vi "WIFI_disconnectOne.vi"(8 "错误输入":errorcluster caption="错误输入（无错误）", 11 "WIFI_Name":string) -> (0 "error out":errorcluster caption="错误输出", 3 "standard output  2":string caption="标准输出")   [LabVIEW 2013]
uses:
  <vilib>/Utility/sysdir.llb/System Directory Type.ctl
panel:
  out "system directory":path caption="系统目录"
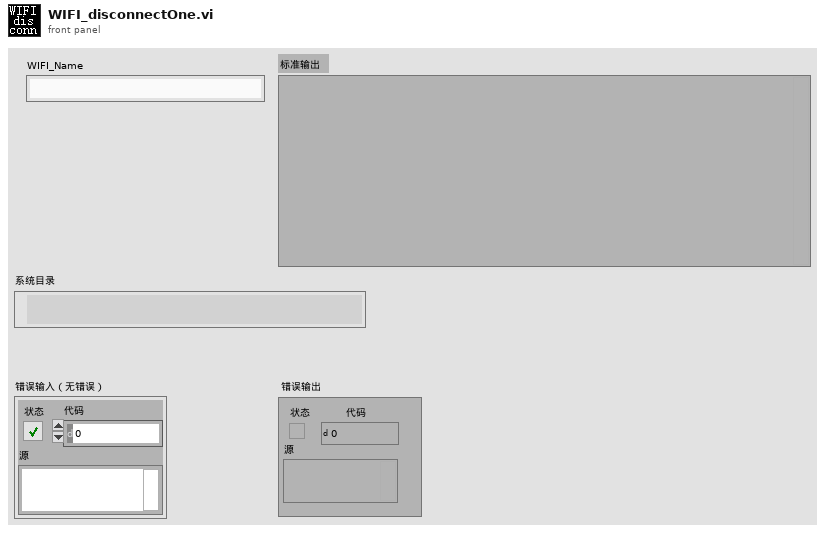
[diagram p1: front panel]
types:
  T1 = typedef "System Directory Type.ctl" = i32
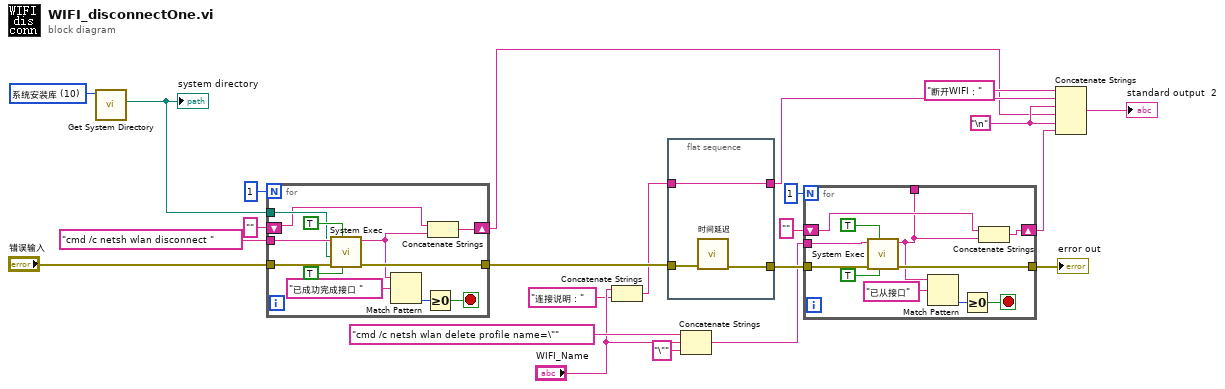
[diagram p0: block diagram]
diagram:
  w10 = "\n"
  w23 = T1 10 items=["用户目录"=0, "用户桌面"=1, "用户文档"=2, "用户应用程序数据"=3, "用户设置"=4, "用户临时目录"=5, "公共文档"=6, "公共应用程序数据"=7, "公共设置"=8, "公共缓存"=13, "系统核心库"=9, "系统安装库"=10, "应用程序文件"=11, "启动盘根目录"=12] ("system directory type")
  n1 = call <vilib>:"Get System Directory.vi"("system directory type"=w23) -> ("system directory"=w19:path)  [unwired: 10 in]
  "system directory" <- w19
  n2 = for {
    N: 1 -> [_]
    tunnel: "cmd /c netsh wlan disconnect " ("command line") -> [w33]
    tunnel: "错误输入" -> [w32]
    tunnel: [w31] -> w20
    tunnel: w19 -> [w30]
    shift-right: [w26] -> w2
    shift-left: "" -> [w25]
    stop <- w27 stop-if-true
    n3 = call <vilib>:"System Exec.vi"("run minimized? (F)"=TRUE, "wait until completion? (T)"=TRUE, "error in (no error)"=w32, "working directory"=w30, "command line"=w33) -> ("error out"=w31:errorcluster, "standard output"=w24:string)  [unwired: 3 in, 2 out]
    n4 = Match Pattern(string=w24, regular expression="已成功完成接口 " ("command line")) -> (offset past match=w28:i32)  [unwired: 1 in, 3 out]
    n5 = Greater Or Equal To 0?(x=w28) -> (x >= 0?=w27:bool)
    n6 = Concatenate Strings(w25, w24) -> (w26:string)
  }
  n7 = Concatenate Strings("WIFI_Name", "连接说明：" ("字符串")) -> (w13:string)
  n8 = flat-sequence {
    tunnel: w20 -> [w38]
    tunnel: [w37] -> w7
    tunnel: [w36] -> w11
    tunnel: w13 -> [w36]
    frame #0 {
      n9 = call "时间延迟"("error in (no error)"=w38) -> ("error out"=w37:errorcluster)  [unwired: 10 in]
    }
  }
  n10 = Concatenate Strings("cmd /c netsh wlan delete profile name=\"" ("command line"), "WIFI_Name", "\"" ("字符串")) -> (w1:string)
  n11 = for {
    N: 1 -> [_]
    tunnel: [w47] -> w8
    tunnel: [w41] -> _
    tunnel: w7 -> [w43]
    shift-right: [w40] -> w4
    shift-left: "" -> [w42]
    tunnel: w1 -> [w39]
    stop <- w44 stop-if-true
    n12 = call <vilib>:"System Exec.vi"("run minimized? (F)"=TRUE, "wait until completion? (T)"=TRUE, "error in (no error)"=w43, "command line"=w39) -> ("error out"=w47:errorcluster, "standard output"=w41:string)  [unwired: 4 in, 2 out]
    n13 = Match Pattern(string=w41, regular expression="已从接口" ("command line")) -> (offset past match=w45:i32)  [unwired: 1 in, 3 out]
    n14 = Greater Or Equal To 0?(x=w45) -> (x >= 0?=w44:bool)
    n15 = Concatenate Strings(w42, w41) -> (w40:string)
  }
  "error out" <- w8
  n16 = Concatenate Strings("断开WIFI：" ("字符串"), w11, w10, w2, w10, w4) -> (→"standard output  2":string)
